vi "Generate Single Chirp.vi"(11 "Signal Configuration":T1={"Chirp Amplitude"=0.1, "I/O Limit"=10.0, "Sample Rate"=1000000.0, "Chirp Duration (s)"=0.01, "Upper Frequency"=0.0, "Lower Frequency"=0.0, "Windowing"=enum."None"}) -> (0 "error out":errorcluster, 1 "dt":dbl, 2 "Number of samples":dbl, 3 "Chirp":waveform(dbl)(graph))   [LabVIEW 2017]
uses:
  controls/Signal Configuration.ctl
  <vilib>/Analysis/4window.llb/Cosine Tapered Window (DBL).vi
  <vilib>/Analysis/4window.llb/Flat Top Window (DBL).vi
  <vilib>/Analysis/4window.llb/Hamming Window (DBL).vi
  <vilib>/Analysis/4window.llb/Hanning Window (DBL).vi
  <vilib>/Analysis/4window.llb/Kaiser-Bessel Window (DBL).vi
  <vilib>/Analysis/4window.llb/Force Window (DBL).vi
  <vilib>/Analysis/4window.llb/AllCosWindow (DBL).vi
  <vilib>/express/express analysis/Spectral/Block/exnSpectralBlock spectral measurements power poly.vi
  <vilib>/express/express analysis/Spectral/Block/exnSpectralBlock spectral measurements power WFM.vi
  <vilib>/ErrorRing/Error Ring.xnode
  <vilib>/express/express analysis/Spectral/XNode/ExpressSpectralMeasurementsBlockNode.xnode
  <vilib>/Analysis/NI_AALPro.lvlib
  <vilib>/Analysis/NI_AALBase.lvlib
panel:
  out "Unwindowed Chirp":waveform(dbl)(graph)
  out "Unwindowed FFT":cluster{"f0":dbl, "df":dbl, "magnitude":dbl[]}(graph)
  out "Windowed FFT":cluster{"f0":dbl, "df":dbl, "magnitude":dbl[]}(graph)
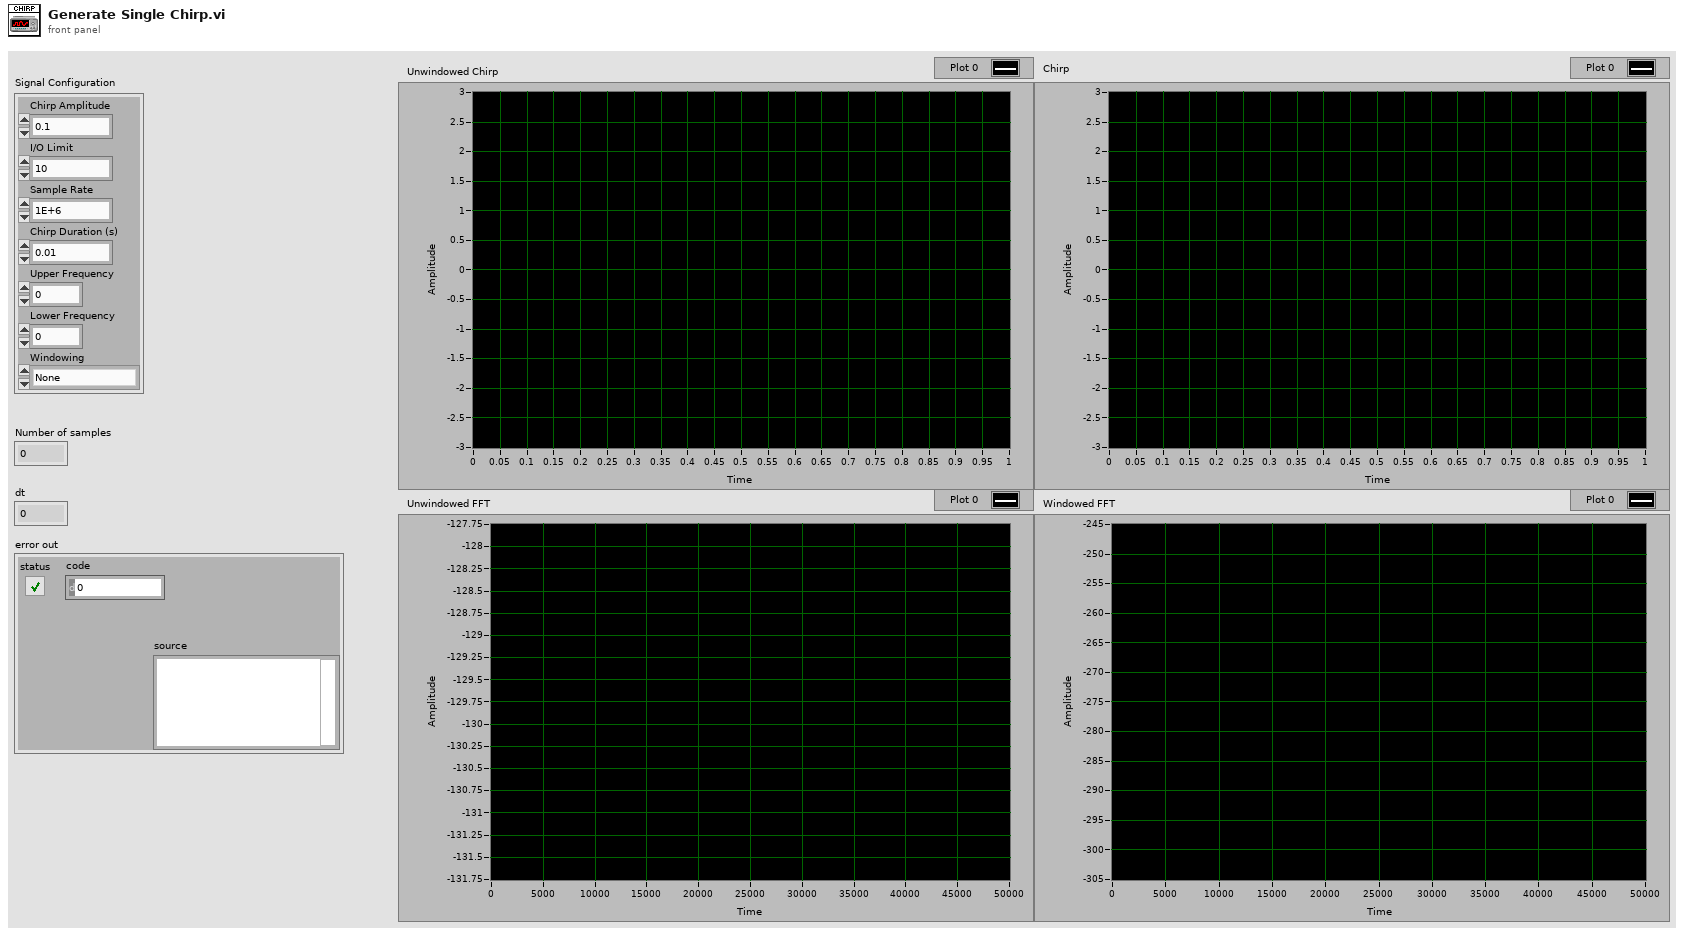
[diagram p1: front panel]
types:
  T1 = typedef "Signal Configuration.ctl" = cluster{"Chirp Amplitude":dbl, "I/O Limit":dbl, "Sample Rate":dbl, "Chirp Duration (s)":dbl, "Upper Frequency":dbl, "Lower Frequency":dbl, "Windowing":enum16{"None", "Exponential", "Flat top", "Hamming", "Hanning", "Kaiser-Bessel", "Rectangular"}}
  T2 = enum16{"None", "Exponential", "Flat top", "Hamming", "Hanning", "Kaiser-Bessel", "Rectangular"}
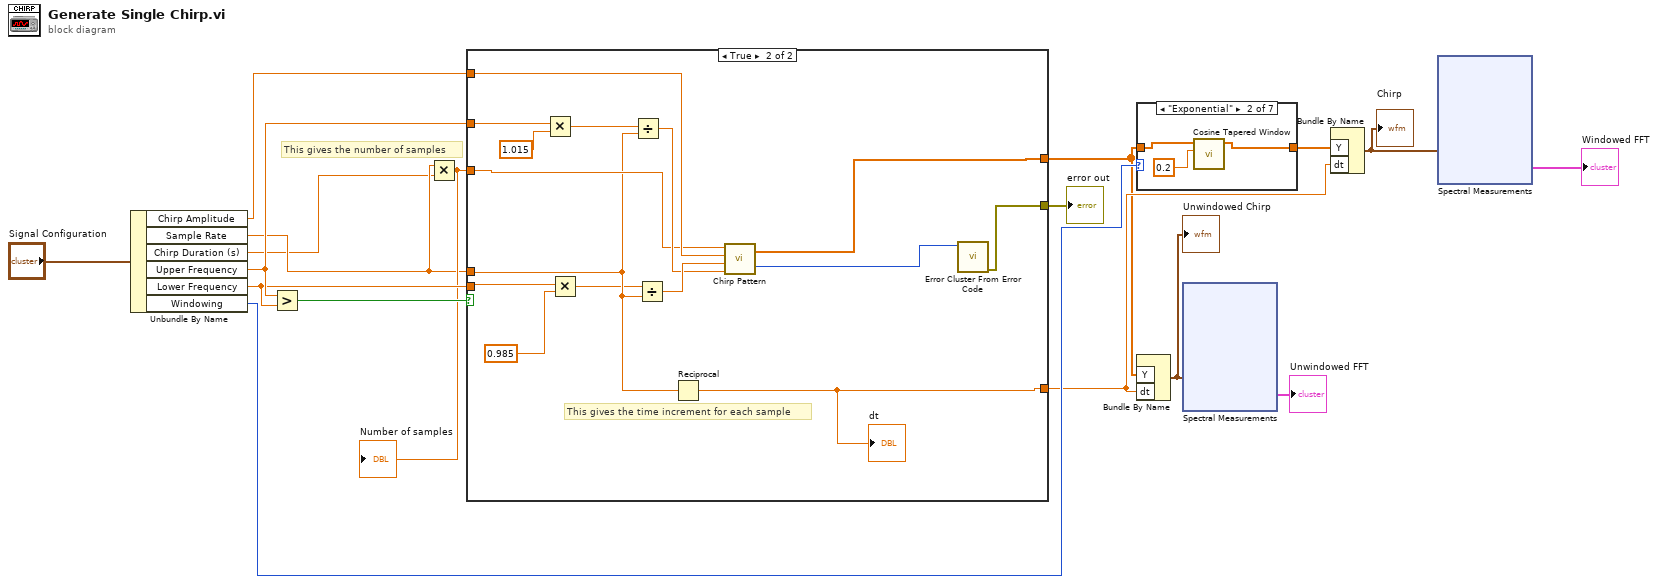
[diagram p0: block diagram]
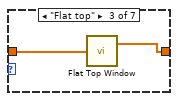
[diagram p3: hidden frame]
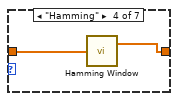
[diagram p4: hidden frame]
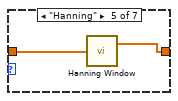
[diagram p5: hidden frame]
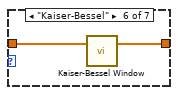
[diagram p6: hidden frame]
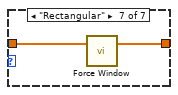
[diagram p7: hidden frame]
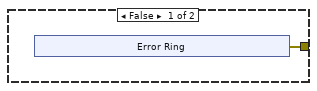
[diagram p8: hidden frame]
diagram:
  # "This gives the number of samples"
  n1 = Unbundle By Name("Signal Configuration") -> ("Chirp Amplitude"=w15:dbl, "Sample Rate"=w2:dbl, "Chirp Duration (s)"=w1:dbl, "Upper Frequency"=w14:dbl, "Lower Frequency"=w13:dbl, "Windowing"=w11:T2)
  n2 = Greater?(x=w14, y=w13) -> (0:w17:bool)
  n3 = Multiply(x=w2, y=w1) -> (x*y=w3:dbl)
  "Number of samples" <- w3
  n4 = case shown="True" w17 {
    tunnel: w14 -> [_ w26]
    tunnel: w13 -> [_ w28]
    tunnel: [w18 w31] -> w16
    tunnel: w2 -> [_ w34]
    tunnel: w3 -> [_ w35]
    tunnel: w15 -> [_ w36]
    tunnel: [_ w33] -> w5
    tunnel: [_ w30] -> w6
    frame False {
      n5 = xnode "Error Ring"() -> ("error out"=w18:errorcluster)
    }
    frame True {
      # "This gives the time increment for each sample"
      n6 = Multiply(x=w26, y=1.015) -> (x*y=w25:dbl)
      n7 = Multiply(x=w28, y=0.985) -> (x*y=w27:dbl)
      n8 = Divide(x=w25, y=w34) -> (x/y=w37:dbl)
      n9 = Divide(x=w27, y=w34) -> (x/y=w38:dbl)
      n10 = Reciprocal(x=w34) -> (1/x=w30:dbl)
      "dt" <- w30
      n11 = call <vilib>:"Chirp Pattern.vi"("f2"=w37, "f1"=w38, "amplitude"=w36, "samples"=w35) -> ("error"=w32:i32, "Chirp Pattern"=w33:dbl[])
      n12 = call <vilib>:"Error Cluster From Error Code.vi"("error code (0)"=w32) -> ("error out"=w31:errorcluster)  [unwired: 8 in]
    }
  }
  "error out" <- w16
  n13 = case shown="\"Exponential\"" w11 {
    tunnel: [w39 w41 w43 w46 w48 w50 w51] -> w10
    tunnel: w5 -> [w39 w42 w44 w45 w47 w49 w52]
    frame "None", Default {
    }
    frame "Exponential" {
      n14 = call-poly <vilib>:"Cosine Tapered Window.vi"("ratio"=0.2, "X"=w42) -> ("Windowed X"=w41:dbl[])  [unwired: 8 in, 1 out]
    }
    frame "Flat top" {
      n15 = call-poly <vilib>:"Flat Top Window.vi"("X"=w44) -> ("Windowed X"=w43:dbl[])  [unwired: 1 out]
    }
    frame "Hamming" {
      n16 = call-poly <vilib>:"Hamming Window.vi"("X"=w45) -> ("Windowed X"=w46:dbl[])  [unwired: 1 out]
    }
    frame "Hanning" {
      n17 = call-poly <vilib>:"Hanning Window.vi"("X"=w47) -> ("Windowed X"=w48:dbl[])  [unwired: 1 out]
    }
    frame "Kaiser-Bessel" {
      n18 = call-poly <vilib>:"Kaiser-Bessel Window.vi"("X"=w49) -> ("Windowed X"=w50:dbl[])  [unwired: 1 in, 1 out]
    }
    frame "Rectangular" {
      n19 = call-poly <vilib>:"Force Window.vi"("X"=w52) -> ("Windowed X"=w51:dbl[])  [unwired: 1 in, 1 out]
    }
  }
  n20 = Bundle By Name("Y"=w5, "dt"=w6) -> (w4:waveform(dbl))  [unwired: 1 in]
  "Unwindowed Chirp" <- w4
  n21 = xnode "Spectral Measurements"("Signals"=w4) -> ("Power Spectrum"=→"Unwindowed FFT":cluster{"f0":dbl, "df":dbl, "magnitude":dbl[]})  [unwired: 1 in, 1 out]
  n22 = Bundle By Name("Y"=w10, "dt"=w6) -> (w9:waveform(dbl))  [unwired: 1 in]
  "Chirp" <- w9
  n23 = xnode "Spectral Measurements"("Signals"=w9) -> ("Power Spectrum"=→"Windowed FFT":cluster{"f0":dbl, "df":dbl, "magnitude":dbl[]})  [unwired: 1 in, 1 out]
